vi "Deploy.vi"(8 "error in (no error)":errorcluster, 9 "Deploy?":bool, 11 "Hatch in":refnum<class "Hatch.lvclass">) -> (0 "error out":errorcluster, 3 "Hatch out":refnum<class "Hatch.lvclass">)   [LabVIEW 2018, in "Hatch.lvlib" / "Hatch.lvclass"]
doc: "Use this VI to either extend or retract the hatch mecanism"
uses:
  Hatch.lvclass
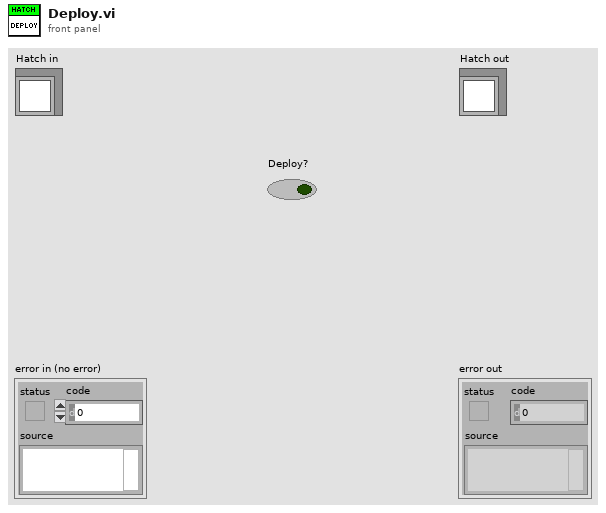
[diagram p1: front panel]
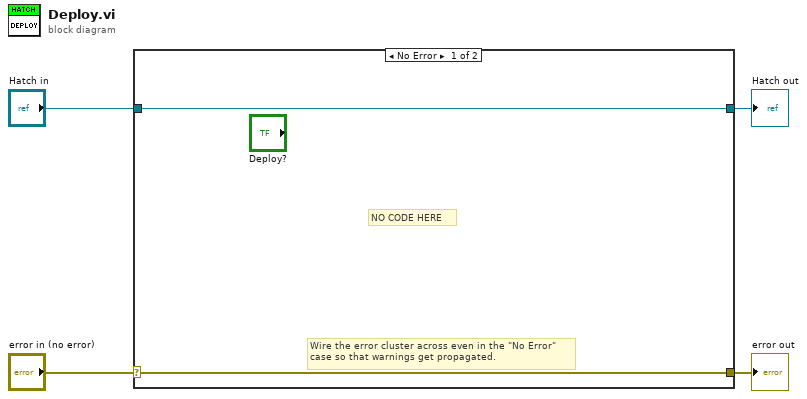
[diagram p0: block diagram]
diagram:
  n1 = case shown="No Error" "error in (no error)" {
    selector: "error in (no error)" -> [w5 w8]
    tunnel: [w5 w8] -> w3
    tunnel: [w6 w7] -> w1
    tunnel: "Hatch in" -> [w6 w7]
    frame No Error {
      # "NO CODE HERE"
      # "Wire the error cluster across even in the \"No Error\"\ncase so that warnings get propagated."
    }
    frame Error {
    }
  }
  "error out" <- w3
  "Hatch out" <- w1
